vi "Pattern Matching (All).vi"() -> ()   [LabVIEW 2014]
doc: "Demonstrate pattern matching algorithms."
uses:
  <vilib>/vision/NI_Vision_Development_Module.lvlib
panel:
  out "Number of Matches Found":i32
  in  "Advanced Options":cluster{"Item":u16, "Value":dbl}[](array[cluster])=[{"Item"=1, "Value"=1.0}, {"Item"=103, "Value"=1.0}] {"Item" items=["LD Sampling - Minimum Constrast"=0, "LD Sampling - Enable Subpixel Accuracy"=1, "LD Sampling - Search Strategy"=2, "LD Sampling - Subpixel Iterations"=3, "LD Sampling - Subpixel Tolerance"=4, "LD Sampling - Initial Match List Length"=5, "LD Sampling - Match List Reduction Factor"=6, "LD Sampling - Initial Step Size"=7, "LD Sampling - Intermediate Angular Accuracy"=8, "-"=9, "Pyramid - Max Pyramid Level"=100, "Pyramid - Minimum Contrast"=102, "Pyramid - Enable Subpixel Accuracy"=103, "Pyramid - Subpixel Iterations"=104, "Pyramid - Subpixel Tolerance"=105, "Pyramid - Initial Match List Length"=106, "Pyramid - Match List Reduction Factor"=107, "Pyramid - Intermediate Angular Accuracy"=108, "Pyramid - Process Border Matches"=109, "Pyramid - Min Match Separation Distance"=111, "Pyramid - Min Match Separation Angle"=112, "Pyramid - Max Match Overlap"=113, "Pyramid - Max Cache in MB"=114, "Pyramid - Clear Cache"=115]}
  in  "Match Parameters":T1={"Number of Matches Requested"=1, "Minimum Match Score"=750.0, "Angle Ranges"=[]} {"Angle Ranges"."End Angle" min=-360 max=360; "Angle Ranges"."Start Angle" min=-360 max=360; "Minimum Match Score" min=0 max=1000; "Number of Matches Requested" min=1 max=9999}
  in  "Algorithm":i32(ring)=2 items=["All", "Low Discrepancy Sampling", "Grayscale Value Pyramid", "Gradients Pyramid"]
  out "Template Report":T2={"Template Contrast"=0, "Grayvalue Max Pyramid Level"=-1, "Grayvalue Optimal Pyramid Level"=-1, "Gradient Max Pyramid Level"=-1, "Gradient Optimal Pyramid Level"=-1}
  in  "Read Next Image":bool
  out "Elapsed Time (ms)":dbl format="%.2f"
  in  "Stop Button":bool
  in  "Match":bool
  in  "Create Template":bool
  out "Template":T3(plugin-control)
  out "Image":T3(plugin-control)
  out "Matches":T4(array[cluster]) {"Bounding Box"."y" format="%.2g"; "Bounding Box"."x" format="%.2g"; "Score" format="%.2f"; "Scale" format="%.2g"; "Angle" format="%.2g"; "Position"."y" format="%.2g"; "Position"."x" format="%.2g"}
  in  "Image File Path":path
  # "Overview: Demonstrate pattern matching algorithms.\nRequirements: Vision Development Module.\nInstructions: \n1. Run the VI.\n2. Click Create Template and select a region of the image.\n3. Click Match."
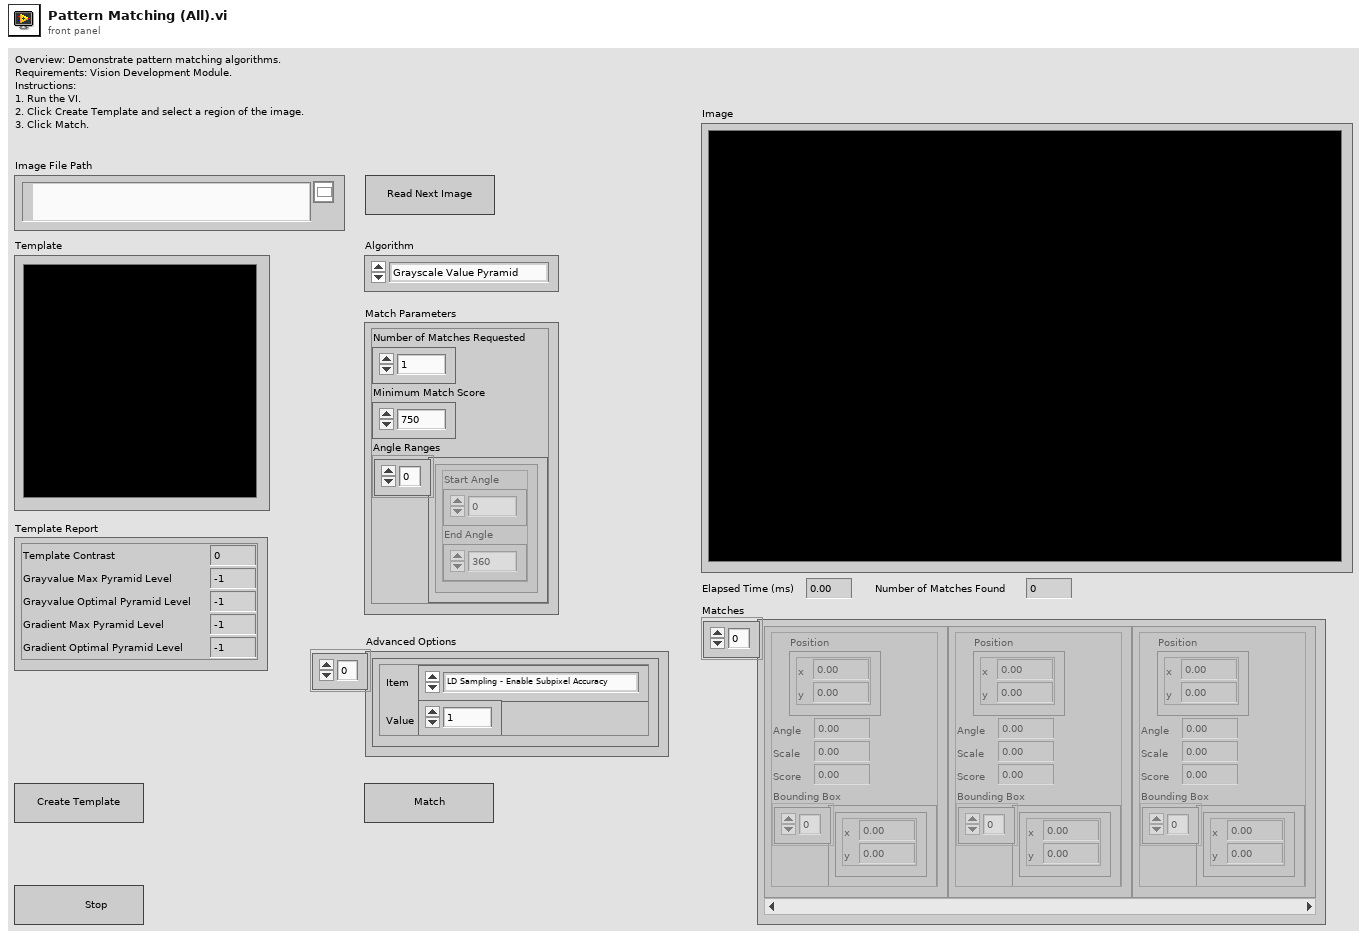
[diagram p1: front panel]
types:
  T1 = cluster{"Number of Matches Requested":i32, "Minimum Match Score":sgl, "Angle Ranges":cluster{"Start Angle":sgl, "End Angle":sgl}[]}
  T2 = cluster{"Template Contrast":i32, "Grayvalue Max Pyramid Level":i32, "Grayvalue Optimal Pyramid Level":i32, "Gradient Max Pyramid Level":i32, "Gradient Optimal Pyramid Level":i32}
  T3 = typedef "IMAQ Image.ctl" = refnum<image>
  T4 = cluster{"Position":cluster{"x":sgl, "y":sgl}, "Angle":sgl, "Scale":sgl, "Score":sgl, "Bounding Box":cluster{"x":sgl, "y":sgl}[]}[]
  T5 = typedef "ROI Descriptor" = cluster{"Global Rectangle":i32[], "Contours":cluster{"ID":enum32{"External", "Internal"}, "Type":u32, "Coordinates":i32[]}[]}
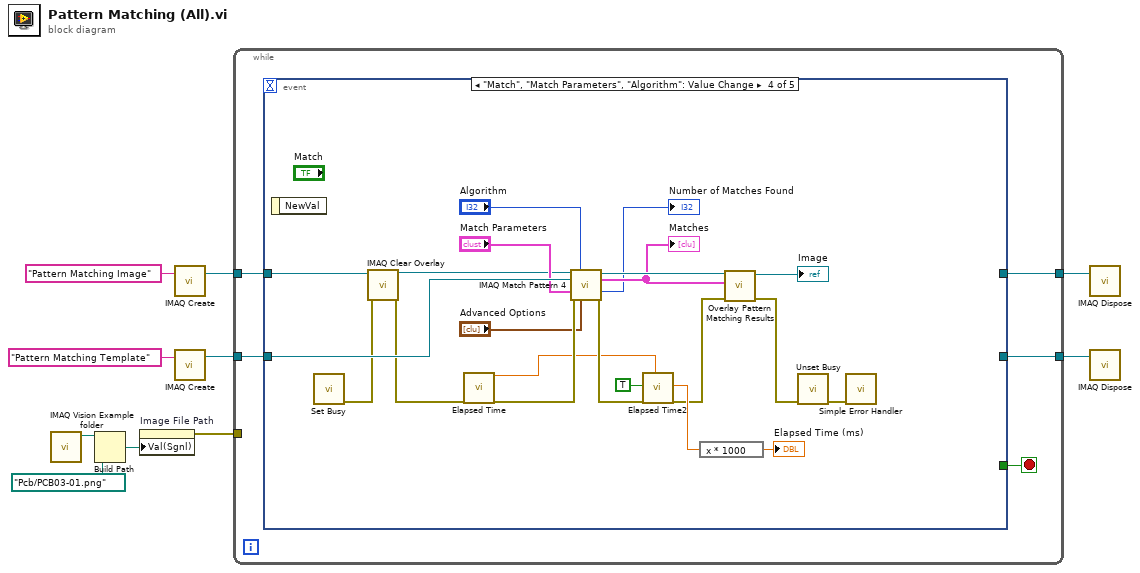
[diagram p0: block diagram]
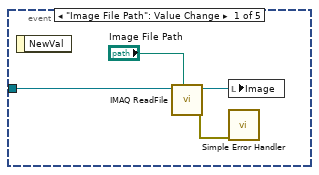
[diagram p2: hidden frame]
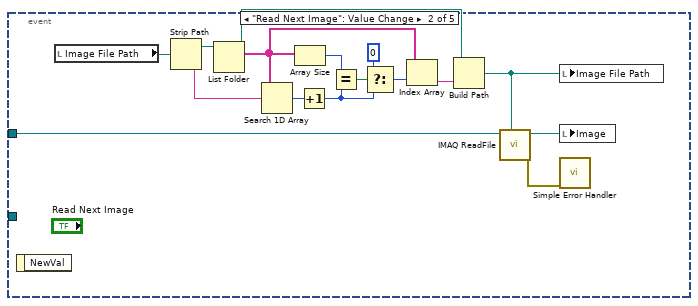
[diagram p3: hidden frame]
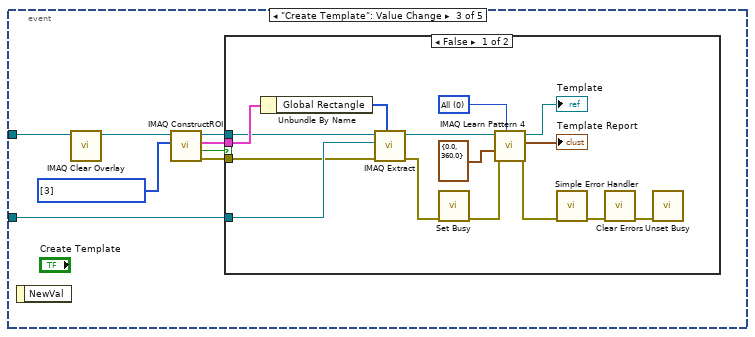
[diagram p4: hidden frame]
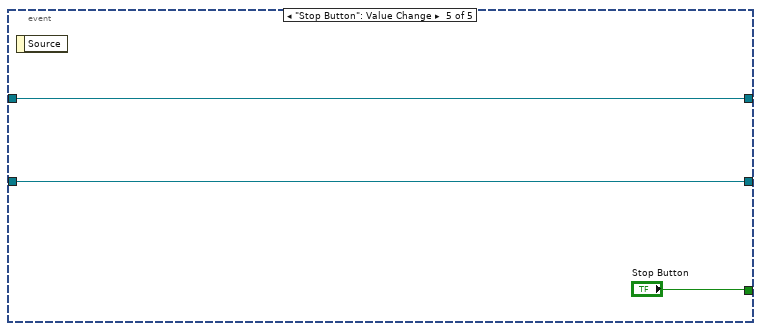
[diagram p6: hidden frame]
diagram:
  n1 = call "IMAQ Vision Example folder.vi"() -> ("Example Image Path"=w7:path)  [unwired: 11 in]
  n2 = Build Path(base path=w7, name or relative path=path "Pcb/PCB03-01.png" ("path out")) -> (appended path=w5:path)
  n3 = property on="Image File Path" class="Path"("Val(Sgnl)"=w5) -> (error out=w8:errorcluster)  [unwired: 2 in, 1 out]
  n4 = call "IMAQ Create"("Image Name"="Pattern Matching Image") -> ("New Image"=w4:T3)  [unwired: 4 in, 1 out]
  n5 = call "IMAQ Create"("Image Name"="Pattern Matching Template") -> ("New Image"=w3:T3)  [unwired: 4 in, 1 out]
  n6 = while {
    tunnel: w8 -> [_]
    tunnel: w4 -> [w14]
    tunnel: w3 -> [w13]
    tunnel: [w12] -> w2
    tunnel: [w11] -> w1
    stop <- w15 stop-if-true
    n7 = event shown="[3] \"Match\", \"Match Parameters\", \"Algorithm\": Value Change" {
      selector: _ -> [_ _ _ _ _]
      dyn-events: _ -> [_ _ _ _ _]
      timeout: _ -> [_ _ _ _ _]
      tunnel: w13 -> [_ _ w39 w79 w80]
      tunnel: w14 -> [w18 w35 w37 w72 w81]
      tunnel: [_ _ _ _ "Stop Button"] -> w15
      tunnel: [_ _ _ _ w81] -> w12
      tunnel: [_ _ _ _ w80] -> w11
      event "Image File Path": Value Change {
        n8 = event-data() -> ()  [unwired: 1 in, 1 out]
        n9 = call "IMAQ ReadFile"("File Path"="Image File Path", "Image"=w18) -> ("error out"=w16:errorcluster, "Image Out"=w17:T3)  [unwired: 5 in, 3 out]
        n10 = local write "Image"(w17) -> ()
        n11 = call <vilib>:"Simple Error Handler.vi"("error in (no error)"=w16) -> ()  [unwired: 4 in, 5 out]
      }
      event "Read Next Image": Value Change {
        n12 = event-data() -> ()  [unwired: 1 in, 1 out]
        n13 = local read "Image File Path"() -> (w33:path)
        n14 = Strip Path(path=w33) -> (stripped path=w32:path, name=w31:string)
        n15 = List Folder(path=w32) -> (path out=w27:path, filenames=w29:string[])  [unwired: 3 in, 2 out]
        n16 = Search 1D Array(1D array=w29, element=w31) -> (index of element=w30:i32)  [unwired: 1 in]
        n17 = Array Size(array=w29) -> (size(s)=w25:i32)
        n18 = Increment(x=w30) -> (x+1=w22:i32)
        n19 = Equal?(x=w25, y=w22) -> (x = y?=w24:bool)
        n20 = Select(t=0 ("x+1"), s=w24, f=w22) -> (s? t:f=w23:i32)
        n21 = Index Array(array=w29, index=w23) -> (element=w28:string)
        n22 = Build Path(base path=w27, name or relative path=w28) -> (appended path=w26:path)
        n23 = call "IMAQ ReadFile"("File Path"=w26, "Image"=w35) -> ("error out"=w20:errorcluster, "Image Out"=w34:T3)  [unwired: 5 in, 3 out]
        n24 = local write "Image File Path"(w26) -> ()
        n25 = local write "Image"(w34) -> ()
        n26 = call <vilib>:"Simple Error Handler.vi"("error in (no error)"=w20) -> ()  [unwired: 4 in, 5 out]
      }
      event "Create Template": Value Change {
        w43 = u32[] [3] items=["No Selection", "Point", "Line", "Rectangle", "Oval", "Polygon", "Freehand Region", "Annulus", "Zoom", "Pan", "Broken Line", "Freehand Line", "Rotated Rectangle"] ("Tools")
        n27 = event-data() -> ()  [unwired: 1 in, 1 out]
        n28 = call "IMAQ Clear Overlay"("Image"=w37) -> ("Image Out"=w36:T3)  [unwired: 9 in, 1 out]
        n29 = call "IMAQ ConstructROI"("Tools"=w43, "Image"=w36) -> ("error out"=w38:errorcluster, "Cancel"=w42:bool, "ROI Descriptor Out"=w40:T5, "Image Out (duplicate)"=w41:T3)  [unwired: 6 in]
        n30 = case shown="False" w42 {
          tunnel: w41 -> [w56 _]
          tunnel: w40 -> [w57 _]
          tunnel: w39 -> [w55 _]
          tunnel: w38 -> [w52 _]
          frame False {
            w53 = 0 items=["All", "Low Discrepancy Sampling", "Grayscale Value Pyramid", "Gradients Pyramid"] ("Algorithm")
            n31 = Unbundle By Name(w57) -> ("Global Rectangle"=w58:i32[])
            n32 = call "IMAQ Extract"("Optional Rectangle"=w58, "error in (no error)"=w52, "Image Dst"=w55, "Image Src"=w56) -> ("error out"=w49:errorcluster, "Image Dst Out"=w54:T3)  [unwired: 6 in]
            n33 = call <vilib>:"Set Busy.vi"("error in (no error)"=w49) -> ("error out"=w48:errorcluster)  [unwired: 9 in, 1 out]
            n34 = call "IMAQ Learn Pattern 4"("Algorithm"=w53, "error in (no error)"=w48, "Angle Range"=cluster{"Start Angle":sgl, "End Angle":sgl} {"Start Angle"=0.0, "End Angle"=360.0}, "Image"=w54) -> ("error out"=w47:errorcluster, "Template Report"=→"Template Report":T2, "Template Image Out"=→"Template":T3)  [unwired: 5 in]
            n35 = call <vilib>:"Simple Error Handler.vi"("error in (no error)"=w47) -> ("error out"=w46:errorcluster)  [unwired: 4 in, 4 out]
            n36 = call <vilib>:"Clear Errors.vi"("error in (no error)"=w46) -> ("error out"=w45:errorcluster)  [unwired: 5 in, 1 out]
            n37 = call <vilib>:"Unset Busy.vi"("error in (no error)"=w45) -> ()  [unwired: 10 in, 1 out]
          }
          frame True {
          }
        }
      }
      event "Match", "Match Parameters", "Algorithm": Value Change {
        n38 = event-data() -> ()  [unwired: 1 in, 1 out]
        n39 = call <vilib>:"Set Busy.vi"() -> ("error out"=w70:errorcluster)  [unwired: 10 in, 1 out]
        n40 = call "IMAQ Clear Overlay"("error in (no error)"=w70, "Image"=w72) -> ("error out"=w67:errorcluster, "Image Out"=w71:T3)  [unwired: 8 in]
        n41 = call "Elapsed Time"("error in (no error)"=w67) -> ("Present (s)"=w62:dbl, "error out"=w66:errorcluster)  [unwired: 11 in, 6 out]
        n42 = call "IMAQ Match Pattern 4"("Image"=w71, "Algorithm"="Algorithm", "Template Image"=w79, "Parameters"="Match Parameters", "error in (no error)"=w66, "Advanced Options"="Advanced Options") -> ("Image (duplicate)"=w76:T3, "Matches (pixel)"=w73:T4, "Number of Matches"=→"Number of Matches Found":i32, "error out"=w65:errorcluster)  [unwired: 5 in, 1 out]
        "Matches" <- w73
        n43 = call "Elapsed Time2"("Reset"=TRUE, "error in (no error)"=w65, "Set Start Time (s)"=w62) -> ("Elapsed Time (s)"=w69:dbl, "error out"=w63:errorcluster)  [unwired: 9 in, 6 out]
        n44 = expression code="x * 1000"(w69) -> (→"Elapsed Time (ms)":dbl)
        n45 = call "Overlay Pattern Matching Results.vi"("error in"=w63, "Matches"=w73, "Image"=w76) -> ("error out"=w74:errorcluster, "Image Out"=→"Image":T3)  [unwired: 7 in]
        n46 = call <vilib>:"Unset Busy.vi"("error in (no error)"=w74) -> ("error out"=w61:errorcluster)  [unwired: 10 in]
        n47 = call <vilib>:"Simple Error Handler.vi"("error in (no error)"=w61) -> ()  [unwired: 4 in, 5 out]
      }
      event "Stop Button": Value Change {
        n48 = event-data() -> ()  [unwired: 1 in, 1 out]
      }
    }
  }
  n49 = call "IMAQ Dispose"("Image"=w2) -> ()  [unwired: 5 in, 1 out]
  n50 = call "IMAQ Dispose"("Image"=w1) -> ()  [unwired: 5 in, 1 out]
